vi "Log Message.vi"(8 "error in (no error)":errorcluster, 11 "Message":string) -> (0 "error out":errorcluster, 3 "logged string":string)   [LabVIEW 2011]
doc: "logs a message to the standard message log, along with a timestamp."
uses:
  2 Globals/2 Message Logger.vi
  Logger.lvclass
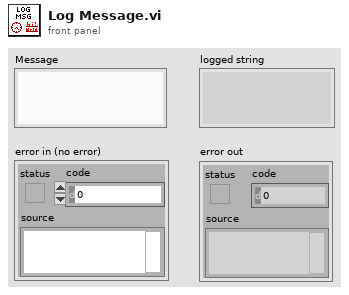
[diagram p1: front panel]
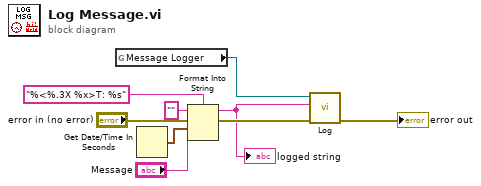
[diagram p0: block diagram]
diagram:
  n1 = global read "2 Message Logger.vi" "Message Logger"() -> (w2:refnum<class "Logger.lvclass">)
  n2 = Get Date/Time In Seconds() -> (seconds since 1Jan1904=w4:timestamp)
  n3 = Format Into String(format string="%<%.3X %x>T: %s" ("initial string"), initial string="", error in="error in (no error)", w4, "Message") -> (resulting string=w5:string, error out=w6:errorcluster)
  "logged string" <- w5
  n4 = call "Log.vi"("error in (no error)"=w6, "Message"=w5, "Logger in"=w2) -> ("error out"=→"error out":errorcluster)  [unwired: 7 in, 1 out]
